vi "parseResetError.vi"(8 "error in (no error)":errorcluster, 10 "DynamicFrameParser":refnum<class "DynamicFrameParser.lvclass">, 11 "ILC in":refnum<class "ILC.lvclass">) -> (0 "error out":errorcluster, 3 "ILC out":refnum<class "ILC.lvclass">)   [LabVIEW 2016, in "RTILC.lvlib" / "ILC.lvclass"]
uses:
  ILC.lvclass
  Common_RT_Modbus/DynamicFrameParser/DynamicFrameParser.lvclass
  ILC.lvclass/ILC.ctl
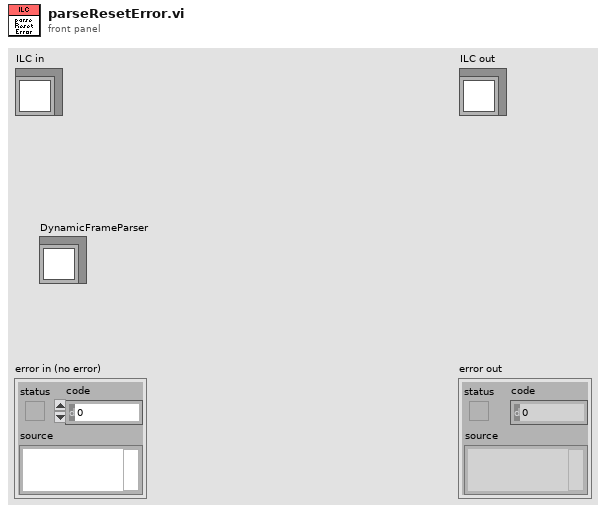
[diagram p1: front panel]
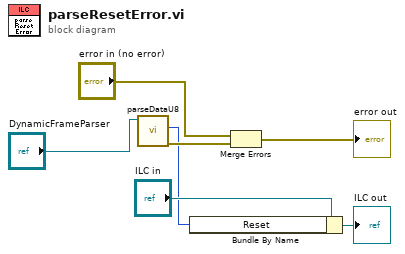
[diagram p0: block diagram]
diagram:
  n1 = call "parseDataU8.vi"("FrameParser in"="DynamicFrameParser") -> ("error out"=w4:errorcluster, "Data"=w1:u8)  [unwired: 8 in, 1 out]
  n2 = Bundle By Name(cluster="ILC in", "Reset"=w1) -> (→"ILC out":refnum<class "ILC.lvclass">)
  n3 = Merge Errors("error in (no error)", w4) -> (→"error out":errorcluster)
